vi "FGV AO PNS.vi"(0 "AO PROP":sgl, 11 "error in (no error)":errorcluster caption="Fehler (Eingang, kein Fehler)", 13 "Aktion":T1) -> (4 "AO PROP":u16, 15 "error out":errorcluster caption="Fehler (Ausgang)")   [LabVIEW 2020, in "PNS.lvlib"]
uses:
  PNS.lvlib
  Aktion FGV AO PNS.ctl
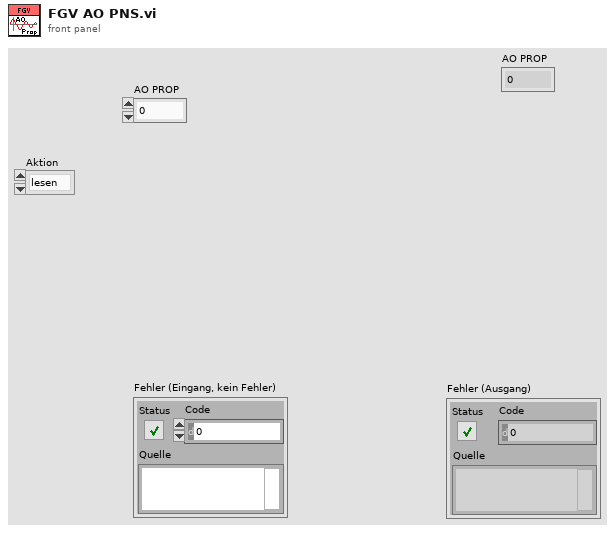
[diagram p1: front panel]
types:
  T1 = typedef "PNS.lvlib/Aktion FGV AO PNS.ctl" = enum16{"lesen", "schreiben"}
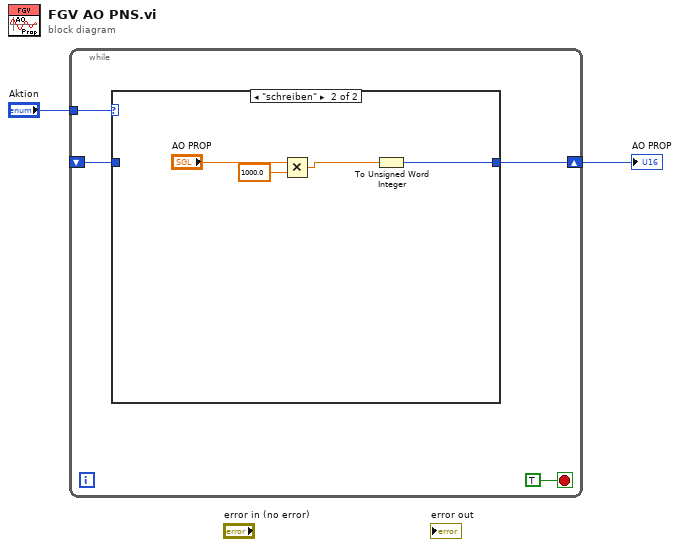
[diagram p0: block diagram]
diagram:
  n1 = while {
    tunnel: "Aktion" -> [w5]
    shift-right: [w4] -> w1
    shift-left: _ -> [w3]
    stop <- TRUE stop-if-true
    n2 = case shown="\"schreiben\"" w5 {
      tunnel: [w7 w8] -> w4
      tunnel: w3 -> [w7 _]
      frame "lesen", Default {
      }
      frame "schreiben" {
        n3 = Multiply(x="AO PROP", y=sgl 1000.0) -> (x*y=w9:sgl)
        n4 = To Unsigned Word Integer(number=w9) -> (unsigned 16bit integer=w8:u16)
      }
    }
  }
  "AO PROP" <- w1
